vi "DS18B20 - 3 devices.vi"() -> ()   [LabVIEW 2013]
uses:
  <vilib>/rvi/Emulation/niFpgaSctlEmulationGetInTimedLoop.vi
  <vilib>/rvi/Emulation/niFpgaEmulationReportErrorSimple.vi
  <vilib>/rvi/Emulation/niFpgaGetClockAttributes.vi
  <vilib>/rvi/Emulation/niFpgaCriticalErrorInLSC.vi
panel:
  in  "stop":bool
  out "Raw Temps":u16[](array[numeric])
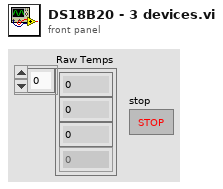
[diagram p1: front panel]
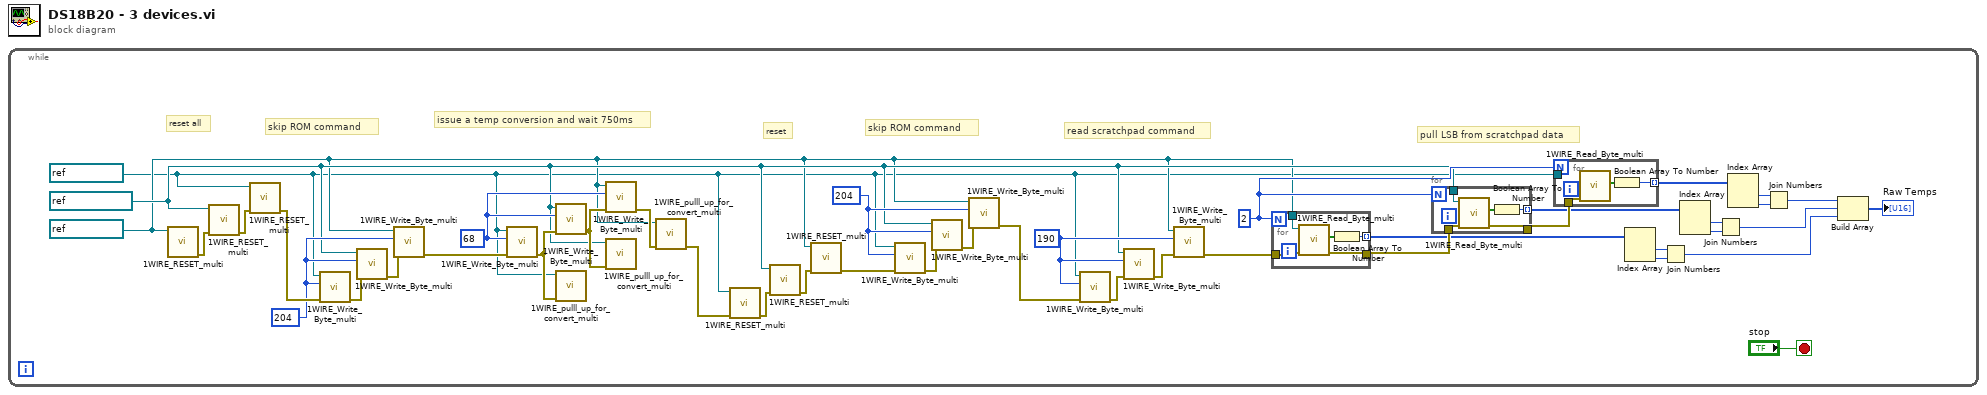
[diagram p0: block diagram]
diagram:
  n1 = while {
    stop <- "stop" stop-if-true
    w1 = refnum<k21> "DS_WIRE" ("FPGA I/O")
    w3 = refnum<k21> "DS_WIRE 1" ("FPGA I/O")
    w2 = refnum<k21> "DS_WIRE" ("FPGA I/O")
    w23 = 2
    w4 = u8 190 ("Tx data 2")
    w28 = u8 204 ("Tx data 2")
    w8 = u8 68 ("Tx data 2")
    w39 = u8 204 ("Tx data 2")
    # "pull LSB from scratchpad data"
    # "read scratchpad command"
    # "skip ROM command"
    # "reset"
    # "issue a temp conversion and wait 750ms"
    # "skip ROM command"
    # "reset all"
    n2 = call "1WIRE_RESET_multi.vi"("FPGA I/O"=w2) -> ("error out"=w43:errorcluster)  [unwired: 9 in, 1 out]
    n3 = call "1WIRE_RESET_multi.vi"("error in"=w43, "FPGA I/O"=w3) -> ("error out"=w42:errorcluster)  [unwired: 8 in, 1 out]
    n4 = call "1WIRE_RESET_multi.vi"("error in"=w42, "FPGA I/O"=w1) -> ("error out"=w41:errorcluster)  [unwired: 8 in, 1 out]
    n5 = call "1WIRE_Write_Byte_multi.vi"("error in"=w41, "Tx data"=w39, "FPGA I/O"=w1) -> ("error out"=w38:errorcluster)  [unwired: 7 in, 1 out]
    n6 = call "1WIRE_Write_Byte_multi.vi"("error in"=w38, "Tx data"=w39, "FPGA I/O"=w3) -> ("error out"=w40:errorcluster)  [unwired: 7 in, 1 out]
    n7 = call "1WIRE_Write_Byte_multi.vi"("error in"=w40, "Tx data"=w39, "FPGA I/O"=w2) -> ("error out"=w10:errorcluster)  [unwired: 7 in, 1 out]
    n8 = call "1WIRE_Write_Byte_multi.vi"("error in"=w10, "Tx data"=w8, "FPGA I/O"=w1) -> ("error out"=w37:errorcluster)  [unwired: 7 in, 1 out]
    n9 = call "1WIRE_Write_Byte_multi.vi"("error in"=w37, "Tx data"=w8, "FPGA I/O"=w3) -> ("error out"=w36:errorcluster)  [unwired: 7 in, 1 out]
    n10 = call "1WIRE_pulll_up_for_convert_multi.vi"("error in"=w37, "FPGA I/O"=w1) -> ()  [unwired: 9 in, 1 out]
    n11 = call "1WIRE_Write_Byte_multi.vi"("error in"=w36, "Tx data"=w8, "FPGA I/O"=w2) -> ("error out"=w35:errorcluster)  [unwired: 7 in, 1 out]
    n12 = call "1WIRE_pulll_up_for_convert_multi.vi"("error in"=w36, "FPGA I/O"=w3) -> ()  [unwired: 9 in, 1 out]
    n13 = call "1WIRE_pulll_up_for_convert_multi.vi"("error in"=w35, "FPGA I/O"=w2) -> ("error out"=w5:errorcluster)  [unwired: 9 in]
    n14 = call "1WIRE_RESET_multi.vi"("error in"=w5, "FPGA I/O"=w1) -> ("error out"=w33:errorcluster)  [unwired: 8 in, 1 out]
    n15 = call "1WIRE_RESET_multi.vi"("error in"=w33, "FPGA I/O"=w3) -> ("error out"=w34:errorcluster)  [unwired: 8 in, 1 out]
    n16 = call "1WIRE_RESET_multi.vi"("error in"=w34, "FPGA I/O"=w2) -> ("error out"=w9:errorcluster)  [unwired: 8 in, 1 out]
    n17 = call "1WIRE_Write_Byte_multi.vi"("error in"=w9, "Tx data"=w28, "FPGA I/O"=w1) -> ("error out"=w30:errorcluster)  [unwired: 7 in, 1 out]
    n18 = call "1WIRE_Write_Byte_multi.vi"("error in"=w30, "Tx data"=w28, "FPGA I/O"=w3) -> ("error out"=w29:errorcluster)  [unwired: 7 in, 1 out]
    n19 = call "1WIRE_Write_Byte_multi.vi"("error in"=w29, "Tx data"=w28, "FPGA I/O"=w2) -> ("error out"=w7:errorcluster)  [unwired: 7 in, 1 out]
    n20 = call "1WIRE_Write_Byte_multi.vi"("error in"=w7, "Tx data"=w4, "FPGA I/O"=w1) -> ("error out"=w31:errorcluster)  [unwired: 7 in, 1 out]
    n21 = call "1WIRE_Write_Byte_multi.vi"("error in"=w31, "Tx data"=w4, "FPGA I/O"=w3) -> ("error out"=w32:errorcluster)  [unwired: 7 in, 1 out]
    n22 = call "1WIRE_Write_Byte_multi.vi"("error in"=w32, "Tx data"=w4, "FPGA I/O"=w2) -> ("error out"=w6:errorcluster)  [unwired: 7 in, 1 out]
    n23 = for {
      N: w23 -> [_]
      tunnel: w6 -> [w56]
      tunnel: [w55] -> w27
      tunnel: [w53] -> w21 mode=indexing
      tunnel: w2 -> [w52]
      n24 = call "1WIRE_Read_Byte_multi.vi"("error in"=w56, "FPGA I/O"=w52) -> ("error out"=w55:errorcluster, "Array"=w54:bool[])  [unwired: 8 in]
      n25 = Boolean Array To Number(Boolean array=w54) -> (number=w53:u8)
    }
    n26 = for {
      N: w23 -> [_]
      tunnel: w3 -> [w47]
      tunnel: w27 -> [w51]
      tunnel: [w50] -> w26
      tunnel: [w48] -> w19 mode=indexing
      n27 = call "1WIRE_Read_Byte_multi.vi"("error in"=w51, "FPGA I/O"=w47) -> ("error out"=w50:errorcluster, "Array"=w49:bool[])  [unwired: 8 in]
      n28 = Boolean Array To Number(Boolean array=w49) -> (number=w48:u8)
    }
    n29 = for {
      N: w23 -> [_]
      tunnel: w1 -> [_]
      tunnel: w26 -> [w46]
      tunnel: [w44] -> w17 mode=indexing
      n30 = call "1WIRE_Read_Byte_multi.vi"("error in"=w46) -> ("Array"=w45:bool[])  [unwired: 9 in, 1 out]
      n31 = Boolean Array To Number(Boolean array=w45) -> (number=w44:u8)
    }
    n32 = Index Array(array=w21) -> (element #1=w16:u8, element #2=w22:u8)  [unwired: 2 in]
    n33 = Join Numbers(hi=w16, lo=w22) -> ((hi.lo)=w11:u16)
    n34 = Index Array(array=w19) -> (element #1=w15:u8, element #2=w20:u8)  [unwired: 2 in]
    n35 = Join Numbers(hi=w15, lo=w20) -> ((hi.lo)=w12:u16)
    n36 = Index Array(array=w17) -> (element #1=w14:u8, element #2=w18:u8)  [unwired: 2 in]
    n37 = Join Numbers(hi=w14, lo=w18) -> ((hi.lo)=w13:u16)
    n38 = Build Array(w13, w12, w11) -> (→"Raw Temps":u16[])
  }
